vi "InsightTelnetComm.vi"(4 "bytes to read":i32=512, 5 "Continue on 6002 Error (FALSE)":bool, 6 "error in":errorcluster, 7 "Timeout, sec":u32=3, 8 "write buffer (\"\")":string, 9 "telnet connection":T1) -> (0 "error out":errorcluster, 2 "response data":string, 3 "telnet  connection out":T1)   [LabVIEW 2015]
uses:
  Telnet Session.ctl
panel:
  out "Bytes Read":i32
  out "On Loop #":i32
  out "Error Code":i32
  out "Written String":string
  out "Response Length":i32
  out "Total Read Lengths":i32
  out "read loop index":i32
  out "return count":i32
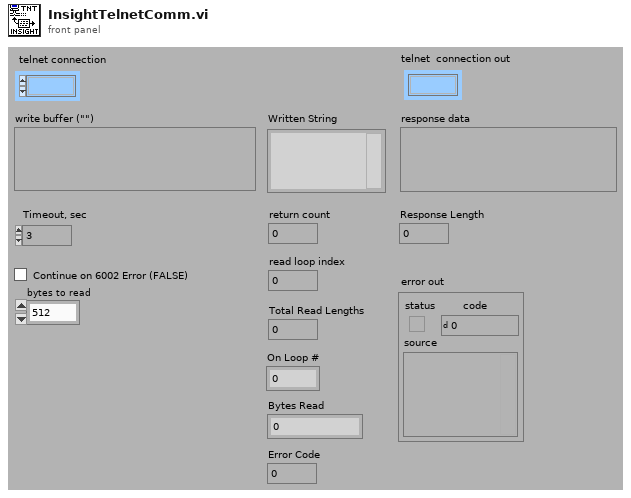
[diagram p1: front panel]
types:
  T1 = typedef "Telnet Session.ctl" = refnum<k1>
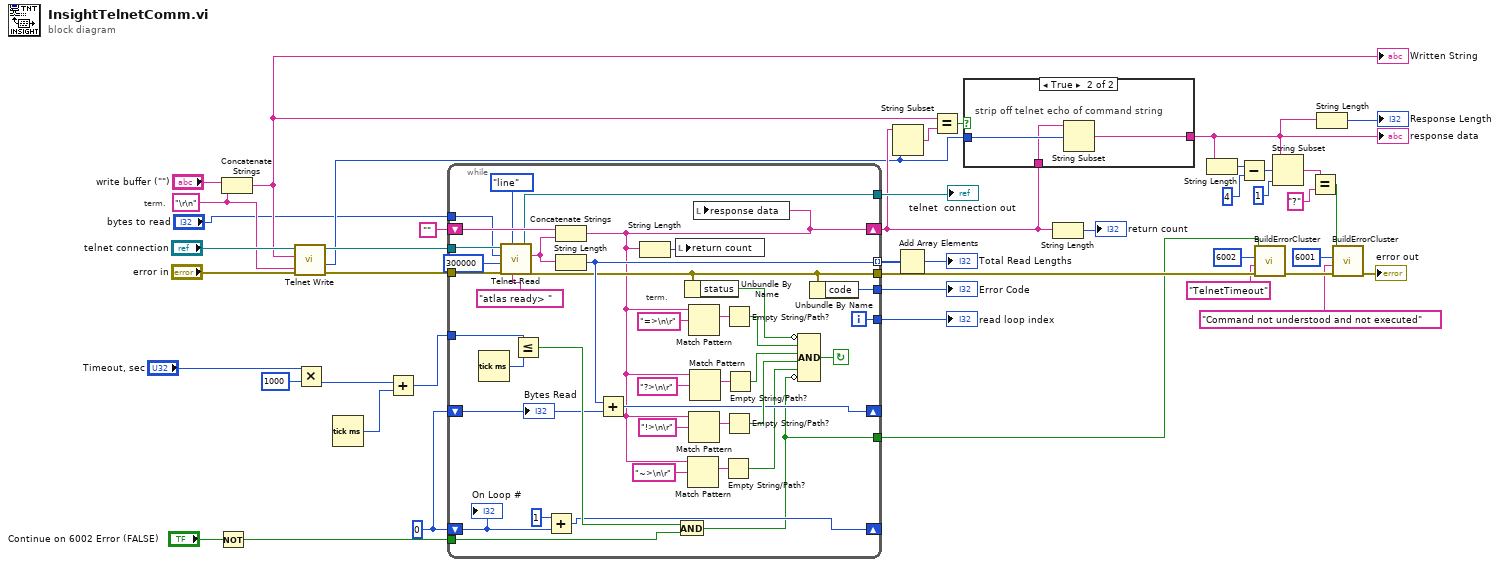
[diagram p0: block diagram]
diagram:
  w9 = 0
  w12 = "\r\n" ("Substring")
  # "term."
  n1 = Not(x="Continue on 6002 Error (FALSE)") -> (.not. x?=w10:bool)
  n2 = Concatenate Strings("write buffer (\"\")", w12) -> (w6:string)
  "Written String" <- w6
  n3 = call "Telnet Write.vi"("line separator (\\n)"=w12, "error in (no error)"="error in", "data in"=w6, "telnet connection"="telnet connection") -> ("error out"=w1:errorcluster, "bytes written"=w3:i32, "telnet  connection out"=w18:T1)  [unwired: 3 in]
  n4 = Multiply(x="Timeout, sec", y=u32 1000) -> (x*y=w41:u32)
  n5 = Tick Count (ms)() -> (millisecond timer value=w40:u32)
  n6 = Add(x=w41, y=w40) -> (x+y=w39:u32)
  n7 = while {
    shift-left: w9 -> [w57]
    shift-right: [w56] -> _
    shift-left: w9 -> [w58]
    shift-right: [w60] -> _
    tunnel: w10 -> [w66]
    tunnel: [w69] -> w13
    tunnel: [w55] -> w16 mode=indexing
    tunnel: [w48] -> w21
    tunnel: [w79] -> w37
    tunnel: [w75] -> w36
    tunnel: [w51] -> w35
    tunnel: w39 -> [w82]
    shift-left: "" -> [w76]
    shift-right: [w46] -> w8
    tunnel: w1 -> [w68]
    tunnel: w18 -> [w64]
    tunnel: "bytes to read" -> [w45]
    i -> [w79]
    stop <- w80 continue-if-true
    # "term."
    n8 = Tick Count (ms)() -> (millisecond timer value=w81:u32)
    n9 = call "Telnet Read.vi"("line separator"="atlas ready> ", "read mode (normal)"=enum16{"normal", "line", "buffered"}."line" ("Method"), "error in (no error)"=w68, "timeout ms (25000)"=300000, "bytes to read"=w45, "telnet connection"=w64) -> ("error out"=w51:errorcluster, "data out"=w54:string, "telnet connection out"=w75:T1)  [unwired: 1 in]
    n10 = Less Or Equal?(x=w82, y=w81) -> (x <= y?=w65:bool)
    n11 = Add(x=1, y=w58) -> (x+y=w60:i32)
    n12 = Concatenate Strings(w76, w54) -> (w46:string)
    n13 = String Length(string=w54) -> (length=w55:i32)
    n14 = Add(x=w55, y=w57) -> (x+y=w56:i32)
    n15 = String Length(string=w46) -> (length=w53:i32)
    n16 = local write "return count"(w53) -> ()
    n17 = And(x=w65, y=w66) -> (x .and. y?=w48:bool)
    n18 = Unbundle By Name(w51) -> ("status"=w67:bool)
    n19 = Match Pattern(string=w46, regular expression="~>\n\r") -> (match substring=w50:string)  [unwired: 1 in, 3 out]
    n20 = Match Pattern(string=w46, regular expression="=>\n\r") -> (match substring=w72:string)  [unwired: 1 in, 3 out]
    n21 = Match Pattern(string=w46, regular expression="!>\n\r") -> (match substring=w71:string)  [unwired: 1 in, 3 out]
    n22 = Match Pattern(string=w46, regular expression="?>\n\r") -> (match substring=w70:string)  [unwired: 1 in, 3 out]
    n23 = local write "response data"(w46) -> ()
    n24 = Empty String/Path?(string/path=w50) -> (empty?=w47:bool)
    n25 = Empty String/Path?(string/path=w72) -> (empty?=w52:bool)
    n26 = Empty String/Path?(string/path=w71) -> (empty?=w73:bool)
    n27 = Empty String/Path?(string/path=w70) -> (empty?=w74:bool)
    n28 = Compound Arithmetic op=AND(invert w67, w52, w74, w73, w47, invert w48) -> (w80:bool)
    n29 = Unbundle By Name(w51) -> ("code"=w69:i32)
    "On Loop #" <- w58
    "Bytes Read" <- w57
  }
  "telnet  connection out" <- w36
  "read loop index" <- w37
  "Error Code" <- w13
  n30 = String Subset(string=w8, length (rest)=w3) -> (substring=w7:string)  [unwired: 1 in]
  n31 = Add Array Elements(numeric array=w16) -> (sum=→"Total Read Lengths":i32)
  n32 = Equal?(x=w6, y=w7) -> (x = y?=w4:bool)
  n33 = case shown="True" w4 {
    tunnel: [w84 w87] -> w5
    tunnel: w3 -> [_ w86]
    tunnel: w8 -> [w84 w85]
    frame False {
    }
    frame True {
      # "strip off telnet echo of command string"
      n34 = String Subset(string=w85, offset (0)=w86) -> (substring=w87:string)  [unwired: 1 in]
    }
  }
  "response data" <- w5
  n35 = String Length(string=w8) -> (length=→"return count":i32)
  n36 = String Length(string=w5) -> (length=w28:i32)
  n37 = Subtract(x=w28, y=4) -> (x-y=w26:i32)
  n38 = call "BuildErrorCluster.vi"("error in (no error)"=w35, "ErrorDescription"="TelnetTimeout", "ErrorCode"=6002, "ErrorStatus"=w21) -> ("error out"=w32:errorcluster)  [unwired: 4 in]
  n39 = String Subset(string=w5, offset (0)=w26, length (rest)=1 ("y")) -> (substring=w24:string)
  n40 = Equal?(x=w24, y="?") -> (x = y?=w22:bool)
  n41 = String Length(string=w5) -> (length=→"Response Length":i32)
  n42 = call "BuildErrorCluster.vi"("error in (no error)"=w32, "ErrorDescription"="Command not understood and not executed", "ErrorCode"=6001, "ErrorStatus"=w22) -> ("error out"=→"error out":errorcluster)  [unwired: 4 in]
